vi "Read Serial Configuration.vi"(8 "error in (no error)":errorcluster, 11 "Plugin_UI in":refnum<class "Plugin_UI.lvclass">) -> (0 "error out":errorcluster, 2 "Hardware Setup":T1={"VISA"="", "Interface Type"=0, "Serial Interface"={"Baud Rate"=19200, "Data Bits "=8, "Parity"=enum."None", "Stop Bits"=0}, "Slave Address"=1} {"Interface Type" items=["GPIB"=1, "VXI"=2, "GPIB-VXI"=3, "Serial"=4, "PXI"=5, "TCPIP"=6, "USB"=7, "FireWire"=9, "Invalid"=0]; "Serial Interface"."Stop Bits" items=["1.0", "1.5", "2.0"]; "Serial Interface"."Baud Rate" items=["1200"=1200, "2400"=2400, "4800"=4800, "9600"=9600, "19200"=19200, "38400"=38400, "57600"=57600, "115200"=115200]; "Slave Address" format="%.0x"}, 3 "Plugin_UI out":refnum<class "Plugin_UI.lvclass">)   [LabVIEW 2020, in "Plugin.lvlib" / "Plugin_UI.lvclass"]
doc: "Read Serial Configuration"
uses:
  Plugin_UI.lvclass
  Serial Configuration.ctl
  builds/Libraries/Shared GUI Library.lvlibp/Shared GUI Library/Instrument Settings/Interface/Interface Type.ctl
  builds/Libraries/Shared GUI Library.lvlibp/Shared GUI Library/Instrument Settings/Interface/Serial Interafce.ctl
  Plugin_UI.lvclass/Plugin_UI.ctl
  builds/Libraries/Shared GUI Library.lvlibp
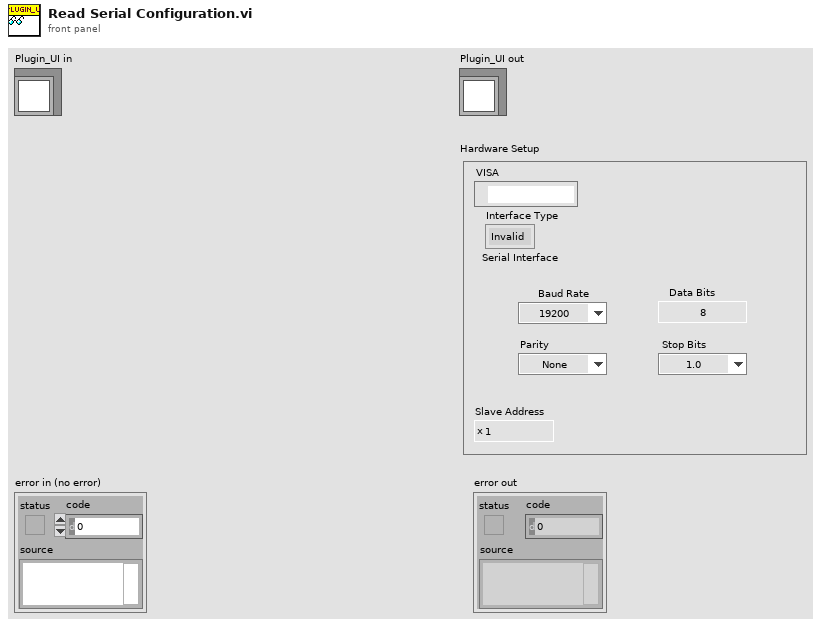
[diagram p1: front panel]
types:
  T1 = typedef "Plugin.lvlib/Plugin_UI.lvclass/Serial Configuration.ctl" = cluster{"VISA":refnum<visa-resource-name>, "Interface Type":T2, "Serial Interface":T3, "Slave Address":u8}
  T2 = typedef "Shared GUI Library.lvlibp/Interface Type.ctl" = u16
  T3 = typedef "Shared GUI Library.lvlibp/Serial Interafce.ctl" = cluster{"Baud Rate":u32, "Data Bits ":u16, "Parity":enum16{"None", "Odd", "Even"}, "Stop Bits":u16}
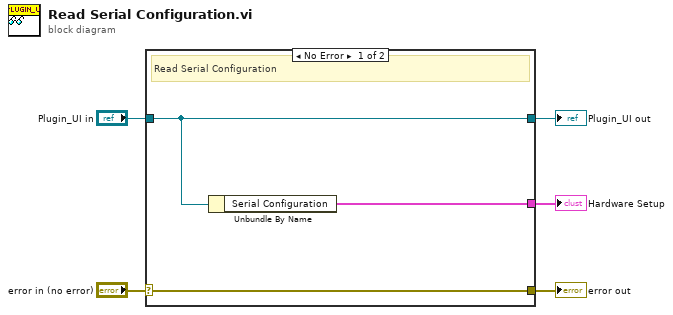
[diagram p0: block diagram]
diagram:
  n1 = case shown="No Error" "error in (no error)" {
    selector: "error in (no error)" -> [w8 w9]
    tunnel: [w8 w9] -> w4
    tunnel: [w7 w10] -> w2
    tunnel: "Plugin_UI in" -> [w7 w10]
    tunnel: [w6 _] -> w1
    frame No Error {
      # "Read Serial Configuration"
      n2 = Unbundle By Name(w7) -> ("Serial Configuration"=w6:T1)
    }
    frame Error {
    }
  }
  "error out" <- w4
  "Plugin_UI out" <- w2
  "Hardware Setup" <- w1
